vi "Launch Sys Cfgs.vi"(8 "error in (no error)":errorcluster, 11 "[V] Sys Cfg Main in":refnum<class "[V] Sys Cfg Main.lvclass">) -> (0 "error out":errorcluster, 3 "[V] Sys Cfg Main out":refnum<class "[V] Sys Cfg Main.lvclass">)   [LabVIEW 2023, in "[V] Sys Cfg Main.lvlib" / "[V] Sys Cfg Main.lvclass"]
uses:
  [V] Sys Cfg Main.lvclass
  [V] Sys Cfg Main.lvclass/[V] Sys Cfg Main.ctl
  <vilib>/ActorFramework/Actor/Actor.lvclass
  [V] Sys Cfg Base/[V] Sys Cfg Base/[V] Sys Cfg Base.lvclass
  C:/Program Files (x86)/National Instruments/LabVIEW 2023/vi.lib/ActorFramework/Actor/Actor.lvclass
  D:/03 GitHub/LabVIEW-System-Config/[V] Sys Cfg Base/[V] Sys Cfg Base/[V] Sys Cfg Base.lvclass
  D:/03 GitHub/LabVIEW-System-Config/[V] Sys Cfg Main/[V] Sys Cfg Main/[V] Sys Cfg Main.lvclass
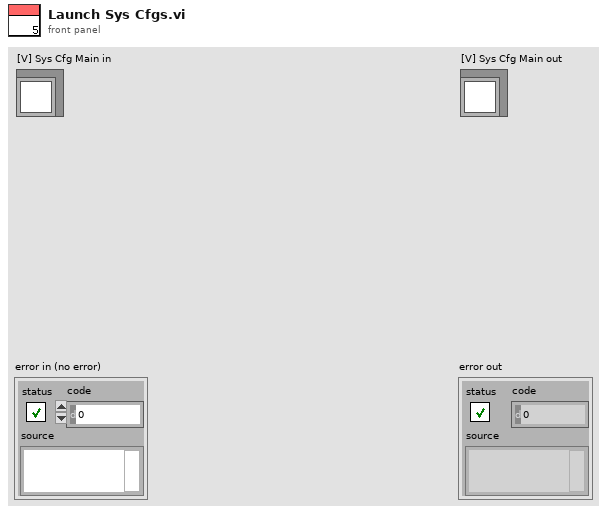
[diagram p1: front panel]
types:
  T1 = map{string, refnum<class "Message Enqueuer.lvclass">}
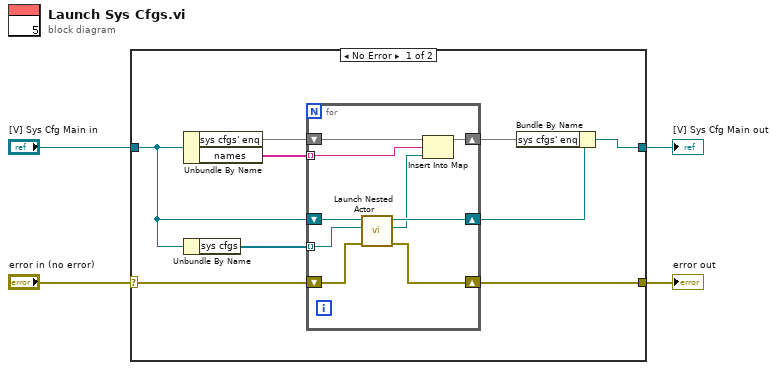
[diagram p0: block diagram]
diagram:
  n1 = case shown="No Error" "error in (no error)" {
    selector: "error in (no error)" -> [w12 w24]
    tunnel: [w5 w24] -> w3
    tunnel: [w8 w23] -> w1
    tunnel: "[V] Sys Cfg Main in" -> [w11 w23]
    frame No Error {
      n2 = Unbundle By Name(w11) -> ("sys cfgs' enq"=w10:T1, "names"=w6:string[])
      n3 = Unbundle By Name(w11) -> ("sys cfgs"=w13:refnum<class "[V] Sys Cfg Base.lvclass">[])
      n4 = for {
        shift-right: [w18] -> w7
        shift-left: w11 -> [w22]
        tunnel: w13 -> [w21] mode=indexing
        shift-right: [w19] -> w5
        shift-left: w12 -> [w20]
        tunnel: w6 -> [w14] mode=indexing
        shift-right: [w16] -> w9
        shift-left: w10 -> [w17]
        n5 = call <vilib>:"Launch Nested Actor.vi"("error in (no error)"=w20, "Nested Actor"=w21, "Caller Actor in"=w22) -> ("error out"=w19:errorcluster, "Nested Actor's Enqueuer"=w15:refnum<class "Message Enqueuer.lvclass">, "Caller Actor out"=w18:refnum<class "[V] Sys Cfg Main.lvclass">)  [unwired: 6 in]
        n6 = Insert Into Map(map in=w17, key=w14, value=w15) -> (map out=w16:T1)  [unwired: 2 out]
      }
      n7 = Bundle By Name(cluster=w7, "sys cfgs' enq"=w9) -> (w8:refnum<class "[V] Sys Cfg Main.lvclass">)
    }
    frame Error {
    }
  }
  "error out" <- w3
  "[V] Sys Cfg Main out" <- w1
